vi "Execute.vi"(6 "WhereIGetMyInformationDescription":string, 8 "error in (no error)":errorcluster caption="Fehler (Eingang, kein Fehler)", 9 "WhereIGetMyInformation":string, 10 "WhoIAm":string, 11 "ApllicationLoadAndConfigurationClass Eingang":refnum<class "LoadConfigurationCsvBased.lvclass"> caption="DNL_LabVIEW Object in") -> (0 "error out":errorcluster caption="Fehler (Ausgang)", 2 "LvDictionary.lvlib:DictionaryString.lvclass":refnum<class "DictionaryString.lvclass">, 3 "ApllicationLoadAndConfigurationClass Ausgang":refnum<class "LoadConfigurationCsvBased.lvclass"> caption="DNL_LabVIEW Object out")   [LabVIEW 2013, in "LoadConfigurationCsvBased.lvclass"]
uses:
  LoadConfigurationCsvBased.lvclass
  LvDictionary/DictionaryStringClass/DictionaryString.lvclass
  <vilib>/Utility/file.llb/Read From Spreadsheet File (string).vi
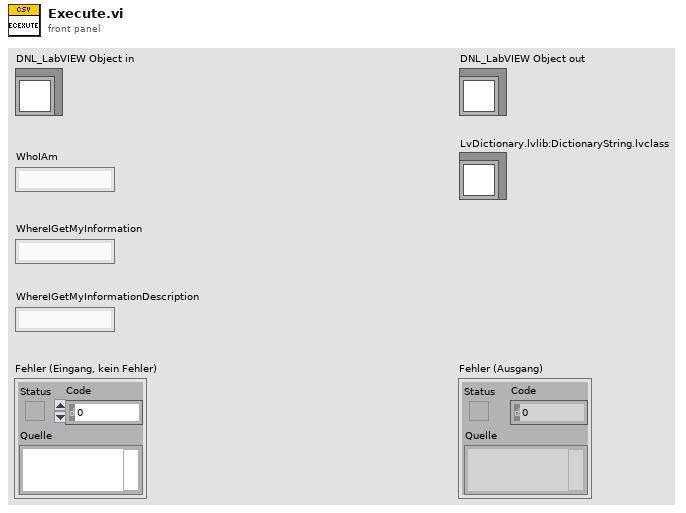
[diagram p1: front panel]
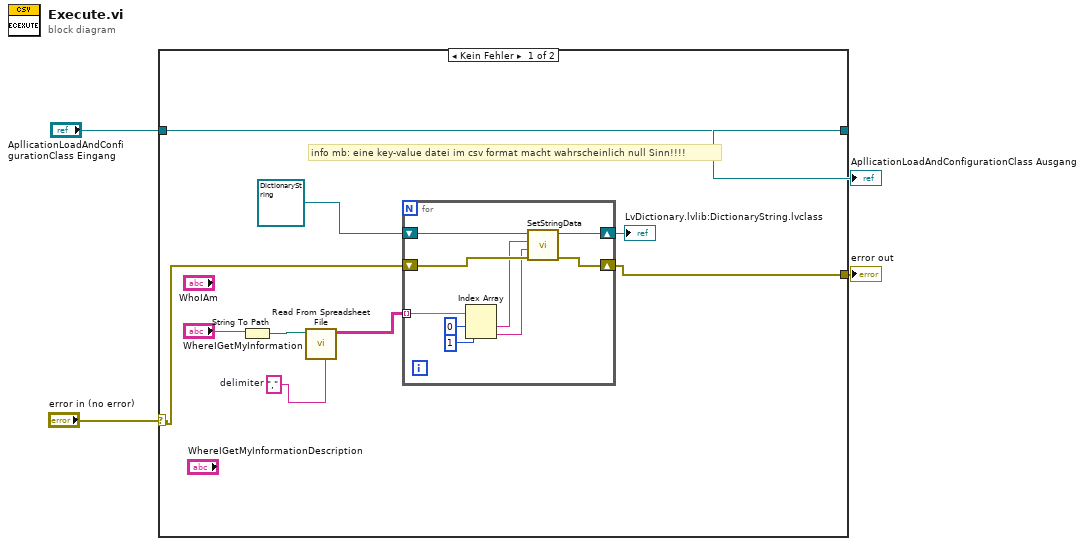
[diagram p0: block diagram]
diagram:
  n1 = case shown="Kein Fehler" "error in (no error)" {
    selector: "error in (no error)" -> [w9 w23]
    tunnel: "ApllicationLoadAndConfigurationClass Eingang" -> [w13 w24]
    tunnel: [w13 w24] -> w2
    tunnel: [w8 w23] -> w1
    frame No Error {
      w7 = ","  # delimiter
      # "info mb: eine key-value datei im csv format macht wahrscheinlich null Sinn!!!!"
      n2 = String To Path(string="WhereIGetMyInformation") -> (path=w11:path)
      n3 = call-poly <vilib>:"Read From Spreadsheet File.vi"("delimiter (\\t)"=w7, "file path (dialog if empty)"=w11) -> ("all rows"=w10:string[][])  [unwired: 5 in, 4 out]
      n4 = for {
        tunnel: w10 -> [w22] mode=indexing
        shift-right: [w15] -> w5
        shift-left: refnum<class "DictionaryString.lvclass"> refnum ("LvDictionary.lvlib:DictionaryString.lvclass") -> [w19]
        shift-right: [w14] -> w8
        shift-left: w9 -> [w18]
        n5 = Index Array(array=w22, index #1=0 ("Index"), index #2=1 ("Index")) -> (element #1=w17:string, element #2=w16:string)
        n6 = call-dynamic "SetStringData.vi"("error in (no error)"=w18, "Value"=w16, "Name"=w17, "DictionaryString Eingang"=w19) -> ("error out"=w14:errorcluster, "DictionaryString Ausgang"=w15:refnum<class "DictionaryString.lvclass">)  [unwired: 6 in]
      }
      "LvDictionary.lvlib:DictionaryString.lvclass" <- w5
    }
    frame Error {
    }
  }
  "error out" <- w1
  "ApllicationLoadAndConfigurationClass Ausgang" <- w2
